vi "Teleop.vi"(10 "Match Info":T1={"Autonomous Elapsed Seconds"=0.0, "TeleOp Elapsed Seconds"=0.0, "Disabled Elapsed Seconds"=0.0, "Visited Autonomous"=FALSE, "Visited TeleOp"=FALSE, "Visited Disabled"=FALSE, "Autonomous Settings"={"Autonomous Style"=enum."Independent", "VI Refnum"=refnum}}, 11 "Call Context":T2) -> ()   [LabVIEW 2012]
doc: "This VI is called for each TeleOp packet received from the DS where the robot is not disabled. It is often used to read from the joysticks and update I/O or to update setpoints for timed control loops. It should complete and return within 20 milliseconds or it may miss DS packets."
uses:
  <vilib>/Rock Robotics/WPI/DriverStation/WPI_DriverStationDerivedRobotMode.ctl
  <vilib>/Rock Robotics/WPI/DriverStation/WPI_DriverStationMatch Info.ctl
  <vilib>/Rock Robotics/WPI/Relay/WPI_RelayValue.ctl
  Robot Global Data.vi
  <vilib>/Rock Robotics/WPI/Joystick/WPI_JoystickGetSetRefNum.vi
panel:
  in  "Ext Const":dbl=0.5
  in  "Dep Const":dbl=1.0
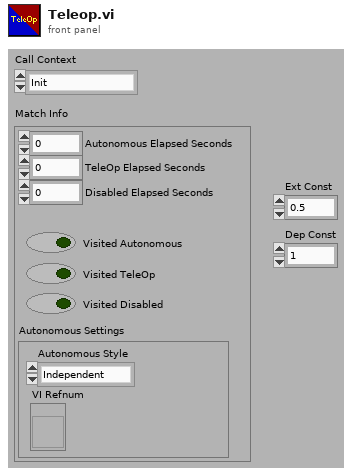
[diagram p1: front panel]
types:
  T1 = typedef "WPI_DriverStationMatch Info.ctl" = cluster{"Autonomous Elapsed Seconds":dbl, "TeleOp Elapsed Seconds":dbl, "Disabled Elapsed Seconds":dbl, "Visited Autonomous":bool, "Visited TeleOp":bool, "Visited Disabled":bool, "Autonomous Settings":cluster{"Autonomous Style":enum16{"Iterative", "Independent"}, "VI Refnum":refnum<vi>}}
  T2 = typedef "WPI_DriverStationDerivedRobotMode.ctl" = enum16{"Init", "Execute", "Stop"}
  T3 = typedef "WPI_RelayValue.ctl" = enum16{"Off", "On", "Forward", "Reverse"}
  T4 = cluster{"Driver Station Digital Input (1-8)[0]":bool, "Driver Station Digital Input (1-8)[1]":bool, "Driver Station Digital Input (1-8)[2]":bool, "Driver Station Digital Input (1-8)[3]":bool, "Driver Station Digital Input (1-8)[4]":bool, "Driver Station Digital Input (1-8)[5]":bool, "Driver Station Digital Input (1-8)[6]":bool, "Driver Station Digital Input (1-8)[7]":bool, "Driver Station Digital Input (1-8)[8]":bool}
  T5 = cluster{"Right Servo High":dbl, "Right Servo Mid":dbl, "Right Servo Low":dbl, "Left Servo High":dbl, "Left Servo Mid":dbl, "Left Servo Low":dbl}
  T6 = typedef "WPI_JoystickDevRef.ctl" = cluster{"Device":T7}
  T7 = typedef "WPI_JoystickDeviceEnum.ctl" = enum16{"USB 1", "USB 2", "USB 3", "USB 4", "Kinect 1", "Kinect 2"}
  T8 = cluster{"axis 1 (x)":dbl, "axis 2 (y)":dbl, "axis 3 (throttle)":dbl, "axis 4":dbl, "axis 5":dbl, "axis 6":dbl}
  T9 = typedef "WPI_RelayDevRef.ctl" = cluster{"DevStatus":errorcluster, "Relay Channel":T10, "Digital Module":T11, "Relay Direction":T12}
  T10 = typedef "FPGA_DIORelayChannel.ctl" = enum8{"Relay 1", "Relay 2", "Relay 3", "Relay 4", "Relay 5", "Relay 6", "Relay 7", "Relay 8", "Invalid"}
  T11 = typedef "FPGA_TypedefDigitalModule.ctl" = enum16{"Digital Module 1", "Digital Module 2"}
  T12 = typedef "WPI_RelayDirection.ctl" = enum16{"Both directions", "Forward only", "Reverse only"}
  T13 = typedef "WPI_ServoDeviceRef.ctl" = cluster{"DeviceStatus":errorcluster, "Digital Module":T11, "PWM Channel":T14, "DeadBand":T15}
  T14 = typedef "FPGA_DIOPWMChannel.ctl" = enum8{"PWM 1", "PWM 2", "PWM 3", "PWM 4", "PWM 5", "PWM 6", "PWM 7", "PWM 8", "PWM 9", "PWM 10", "Invalid"}
  T15 = typedef "WPI_PWMDeadband.ctl" = cluster{"Name":string, "maxPositivePwm":i32, "minPositivePwm":i32, "centerPwm":i32, "maxNegativePwm":i32, "minNegativePwm":i32, "angularRange":u16}
  T16 = typedef "WPI_MotorControlDeviceRef.ctl" = cluster{"DeviceStatus":errorcluster, "Type":enum16{"PWM", "CAN"}, "PWM":cluster{"Digital Module":T11, "PWM Channel":T14, "DeadBand":T15}, "CAN":cluster{"Device Number":u8, "Control Mode":T17, "Semaphore":T18, "Max Vout":dbl}, "Invert":bool, "TransformRef":T19, "InvTransformRef":T19}
  T17 = typedef "WPI_CANJaguar_ControlMode.ctl" = enum8{"Percent VBus", "Current", "Speed", "Position", "Voltage"}
  T18 = typedef "Semaphore RefNum" = refnum<k1>
  T19 = typedef "WPI_PWMTransform_ConPane.ctl" = refnum<vi>
  T20 = typedef "WPI_JoystickButtonState.ctl" = cluster{"Button 1":bool, "Button 2":bool, "Button 3":bool, "Button 4":bool, "Button 5":bool, "Button 6":bool, "Button 7":bool, "Button 8":bool, "Button 9":bool, "Button 10":bool, "Button 11":bool, "Button 12":bool}
  T21 = cluster{"FlipperLeftUp":dbl, "FlipperLeftDown":dbl, "FlipperRightUp":dbl, "FlipperRightDown":dbl, "KickerLeftBack":dbl, "KickerLeftForward":dbl, "KickerRightBack":dbl, "KickerRightForward":dbl}
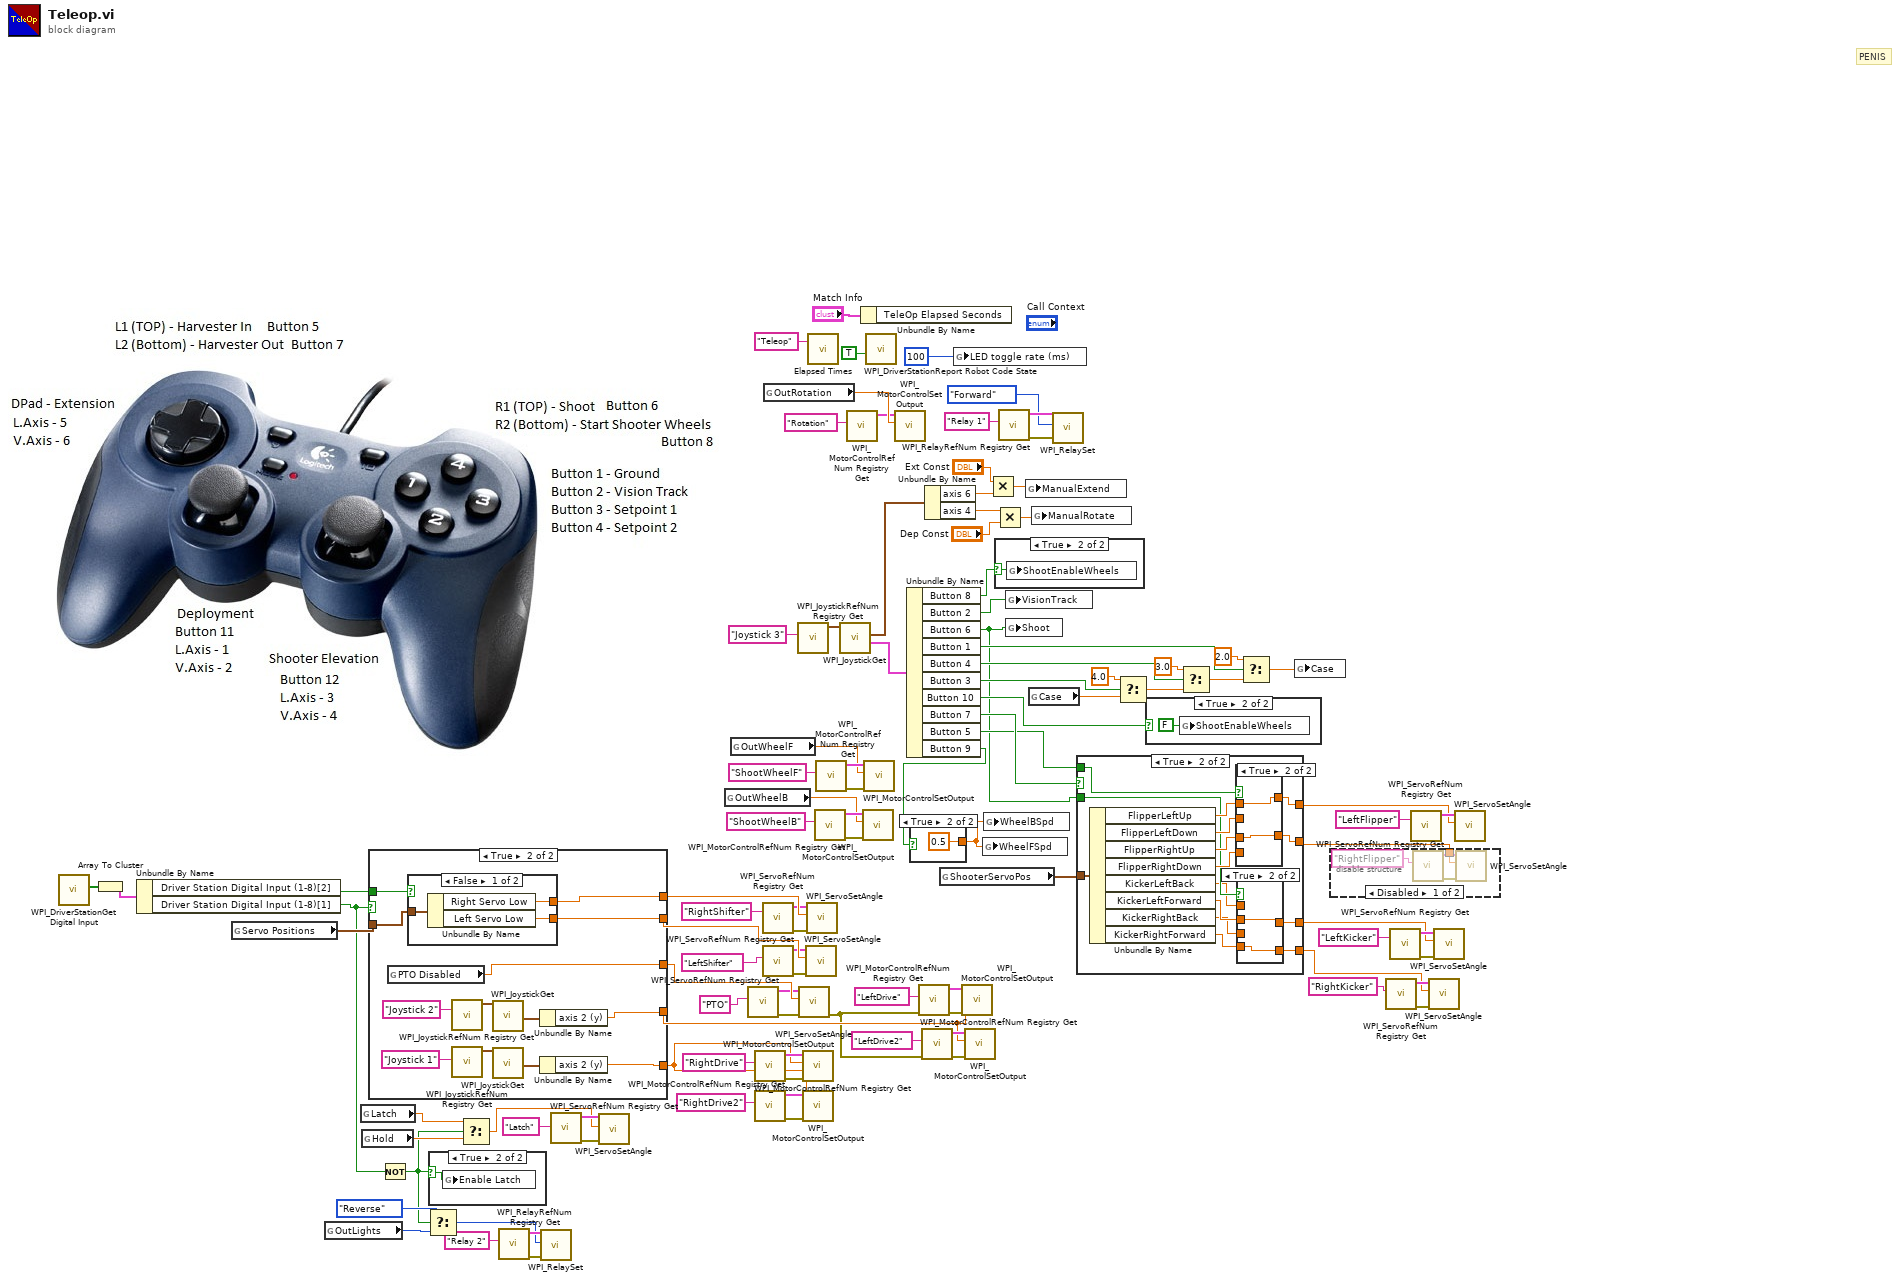
[diagram p0: block diagram]
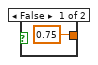
[diagram p2: hidden frame]
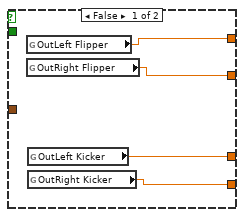
[diagram p4: hidden frame]
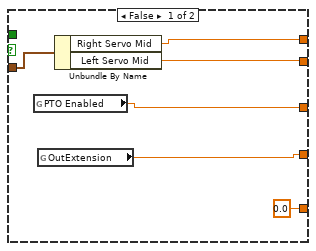
[diagram p8: hidden frame]
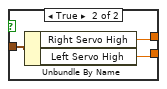
[diagram p9: hidden frame]
diagram:
  # "PENIS"
  n1 = call <vilib>:"WPI_DriverStationGet Digital Input.vi"() -> ("Driver Station Digital Input (1-8)"=w73:bool[])  [unwired: 11 in]
  n2 = Array To Cluster(array=w73) -> (cluster=w72:T4)
  n3 = Unbundle By Name(w72) -> ("Driver Station Digital Input (1-8)[2]"=w71:bool, "Driver Station Digital Input (1-8)[1]"=w32:bool)
  n4 = global read "Robot Global Data.vi" "Servo Positions"() -> (w70:T5)
  n5 = global read "Robot Global Data.vi" "OutLights"() -> (w38:T3)
  n6 = global read "Robot Global Data.vi" "Latch"() -> (w5:dbl)
  n7 = global read "Robot Global Data.vi" "Hold"() -> (w4:dbl)
  n8 = case shown="True" w32 {
    tunnel: w71 -> [_ w124]
    tunnel: w70 -> [w111 w123]
    tunnel: [w110 w122] -> w69
    tunnel: [w109 w121] -> w68
    tunnel: [w108 w120] -> w61
    tunnel: [w106 w113] -> w60
    tunnel: [0.0 w112] -> w59
    frame False {
      n9 = global read "Robot Global Data.vi" "PTO Enabled"() -> (w108:dbl)
      n10 = global read "Robot Global Data.vi" "OutExtension"() -> (w106:dbl)
      n11 = Unbundle By Name(w111) -> ("Right Servo Mid"=w110:dbl, "Left Servo Mid"=w109:dbl)
    }
    frame True {
      n12 = global read "Robot Global Data.vi" "PTO Disabled"() -> (w120:dbl)
      n13 = case shown="False" w124 {
        tunnel: w123 -> [w127 w130]
        tunnel: [w126 w129] -> w122
        tunnel: [w125 w128] -> w121
        frame False {
          n14 = Unbundle By Name(w127) -> ("Right Servo Low"=w126:dbl, "Left Servo Low"=w125:dbl)
        }
        frame True {
          n15 = Unbundle By Name(w130) -> ("Right Servo High"=w129:dbl, "Left Servo High"=w128:dbl)
        }
      }
      n16 = call <vilib>:"WPI_JoystickRefNum Registry Get.vi"("refnum name"="Joystick 2") -> ("JoystickDevRef"=w114:T6)  [unwired: 1 in, 9 out]
      n17 = call <vilib>:"WPI_JoystickRefNum Registry Get.vi"("refnum name"="Joystick 1") -> ("JoystickDevRef"=w118:T6)  [unwired: 1 in, 9 out]
      n18 = call <vilib>:"WPI_JoystickGet.vi"("JoystickDevRef"=w114) -> ("Axes"=w116:T8)  [unwired: 1 in, 5 out]
      n19 = call <vilib>:"WPI_JoystickGet.vi"("JoystickDevRef"=w118) -> ("Axes"=w119:T8)  [unwired: 1 in, 5 out]
      n20 = Unbundle By Name(w116) -> ("axis 2 (y)"=w113:dbl)
      n21 = Unbundle By Name(w119) -> ("axis 2 (y)"=w112:dbl)
    }
  }
  n22 = Not(x=w32) -> (.not. x?=w3:bool)
  n23 = Select(t=WPI_RelayValue."Reverse" ("RelayValue"), s=w3, f=w38) -> (s? t:f=w36:T3)
  n24 = case shown="True" w3 {
    selector: w3 -> [_ w131]
    frame False {
    }
    frame True {
      n25 = global write "Robot Global Data.vi" "Enable Latch"(w131) -> ()
    }
  }
  n26 = Select(t=w5, s=w3, f=w4) -> (s? t:f=w31:dbl)
  n27 = call <vilib>:"WPI_RelayRefNum Registry Get.vi"("refnum name"="Relay 2") -> ("error out"=w44:errorcluster, "RelayDevRef"=w42:T9)  [unwired: 9 in]
  n28 = call <vilib>:"WPI_RelaySet.vi"("error in (no error)"=w44, "RelayValue"=w36, "RelayDevRef"=w42) -> ()  [unwired: 7 in, 2 out]
  n29 = call <vilib>:"WPI_ServoRefNum Registry Get.vi"("refnum name"="Latch") -> ("error out"=w35:errorcluster, "ServoDeviceRef"=w33:T13)  [unwired: 9 in]
  n30 = call <vilib>:"WPI_ServoSetAngle.vi"("error in (no error)"=w35, "Angle"=w31, "ServoDeviceRef"=w33) -> ()  [unwired: 7 in, 2 out]
  n31 = global read "Robot Global Data.vi" "OutWheelB"() -> (w23:dbl)
  n32 = global read "Robot Global Data.vi" "OutWheelF"() -> (w24:dbl)
  n33 = call <vilib>:"WPI_ServoRefNum Registry Get.vi"("refnum name"="PTO") -> ("error out"=w54:errorcluster, "ServoDeviceRef"=w55:T13)  [unwired: 9 in]
  n34 = call <vilib>:"WPI_MotorControlRefNum Registry Get.vi"("refnum name"="RightDrive") -> ("error out"=w83:errorcluster, "MotorControlDevRef"=w85:T16)  [unwired: 9 in]
  n35 = call <vilib>:"WPI_MotorControlRefNum Registry Get.vi"("refnum name"="RightDrive2") -> ("error out"=w76:errorcluster, "MotorControlDevRef"=w74:T16)  [unwired: 9 in]
  n36 = call <vilib>:"WPI_ServoRefNum Registry Get.vi"("refnum name"="RightShifter") -> ("error out"=w64:errorcluster, "ServoDeviceRef"=w65:T13)  [unwired: 9 in]
  n37 = call <vilib>:"WPI_ServoRefNum Registry Get.vi"("refnum name"="LeftShifter") -> ("error out"=w66:errorcluster, "ServoDeviceRef"=w67:T13)  [unwired: 9 in]
  n38 = global read "Robot Global Data.vi" "OutRotation"() -> (w58:dbl)
  n39 = call <vilib>:"WPI_JoystickRefNum Registry Get.vi"("refnum name"="Joystick 3") -> ("JoystickDevRef"=w102:T6)  [unwired: 9 in, 1 out]
  n40 = call <vilib>:"WPI_ServoSetAngle.vi"("error in (no error)"=w54, "Angle"=w61, "ServoDeviceRef"=w55) -> ("error out"=w50:errorcluster)  [unwired: 7 in, 1 out]
  n41 = call <vilib>:"WPI_MotorControlSetOutput.vi"("error in (no error)"=w83, "Output"=w59, "MotorControlDevRef"=w85) -> ()  [unwired: 6 in, 3 out]
  n42 = call <vilib>:"WPI_MotorControlSetOutput.vi"("error in (no error)"=w76, "Output"=w59, "MotorControlDevRef"=w74) -> ()  [unwired: 6 in, 3 out]
  n43 = call <vilib>:"WPI_ServoSetAngle.vi"("error in (no error)"=w66, "Angle"=w68, "ServoDeviceRef"=w67) -> ()  [unwired: 7 in, 2 out]
  n44 = call <vilib>:"WPI_ServoSetAngle.vi"("error in (no error)"=w64, "Angle"=w69, "ServoDeviceRef"=w65) -> ()  [unwired: 7 in, 2 out]
  n45 = call "Elapsed Times.vi"("Call Name"="Teleop") -> ()  [unwired: 2 in, 1 out]
  n46 = call <vilib>:"WPI_MotorControlRefNum Registry Get.vi"("refnum name"="ShootWheelB") -> ("error out"=w26:errorcluster, "MotorControlDevRef"=w27:T16)  [unwired: 9 in]
  n47 = call <vilib>:"WPI_MotorControlRefNum Registry Get.vi"("refnum name"="ShootWheelF") -> ("error out"=w28:errorcluster, "MotorControlDevRef"=w25:T16)  [unwired: 9 in]
  n48 = call <vilib>:"WPI_JoystickGet.vi"("JoystickDevRef"=w102) -> ("Buttons"=w100:T20, "Axes"=w99:T8)  [unwired: 4 in, 1 out]
  n49 = call <vilib>:"WPI_MotorControlRefNum Registry Get.vi"("refnum name"="Rotation") -> ("MotorControlDevRef"=w56:T16)  [unwired: 9 in, 1 out]
  n50 = Unbundle By Name("Match Info") -> ()  [unwired: 1 out]
  n51 = call <vilib>:"WPI_MotorControlSetOutput.vi"("error in (no error)"=w26, "Output"=w23, "MotorControlDevRef"=w27) -> ()  [unwired: 6 in, 3 out]
  n52 = call <vilib>:"WPI_MotorControlSetOutput.vi"("error in (no error)"=w28, "Output"=w24, "MotorControlDevRef"=w25) -> ()  [unwired: 6 in, 3 out]
  n53 = call <vilib>:"WPI_DriverStationReport Robot Code State.vi"("TeleOp"=TRUE ("Autonomous")) -> ()  [unwired: 10 in, 1 out]
  n54 = call <vilib>:"WPI_MotorControlSetOutput.vi"("Output"=w58, "MotorControlDevRef"=w56) -> ()  [unwired: 7 in, 3 out]
  n55 = Unbundle By Name(w100) -> ("Button 8"=w87:bool, "Button 2"=w98:bool, "Button 6"=w7:bool, "Button 1"=w97:bool, "Button 4"=w95:bool, "Button 3"=w94:bool, "Button 10"=w22:bool, "Button 7"=w21:bool, "Button 5"=w20:bool, "Button 9"=w1:bool)
  n56 = case shown="True" w1 {
    tunnel: [0.75 0.5] -> w2
    frame False {
    }
    frame True {
    }
  }
  n57 = call <vilib>:"WPI_MotorControlRefNum Registry Get.vi"("error in (no error)"=w50, "refnum name"="LeftDrive") -> ("error out"=w78:errorcluster, "MotorControlDevRef"=w81:T16)  [unwired: 8 in]
  n58 = call <vilib>:"WPI_MotorControlRefNum Registry Get.vi"("error in (no error)"=w50, "refnum name"="LeftDrive2") -> ("error out"=w77:errorcluster, "MotorControlDevRef"=w79:T16)  [unwired: 8 in]
  n59 = Unbundle By Name(w99) -> ("axis 6"=w41:dbl, "axis 4"=w51:dbl)
  n60 = global read "Robot Global Data.vi" "ShooterServoPos"() -> (w8:T21)
  n61 = global write "Robot Global Data.vi" "LED toggle rate (ms)"(u32 100 ("LED ms toggle rate")) -> ()
  n62 = call <vilib>:"WPI_MotorControlSetOutput.vi"("error in (no error)"=w78, "Output"=w60, "MotorControlDevRef"=w81) -> ()  [unwired: 6 in, 3 out]
  n63 = call <vilib>:"WPI_MotorControlSetOutput.vi"("error in (no error)"=w77, "Output"=w60, "MotorControlDevRef"=w79) -> ()  [unwired: 6 in, 3 out]
  n64 = global write "Robot Global Data.vi" "WheelFSpd"(w2) -> ()
  n65 = global write "Robot Global Data.vi" "WheelBSpd"(w2) -> ()
  n66 = Multiply(x="Ext Const", y=w41) -> (x*y=w39:dbl)
  n67 = Multiply(x=w51, y="Dep Const") -> (x*y=w49:dbl)
  n68 = case shown="True" w87 {
    selector: w87 -> [_ w134]
    frame False {
    }
    frame True {
      n69 = global write "Robot Global Data.vi" "ShootEnableWheels"(w134) -> ()
    }
  }
  n70 = call <vilib>:"WPI_RelayRefNum Registry Get.vi"("refnum name"="Relay 1") -> ("error out"=w46:errorcluster, "RelayDevRef"=w48:T9)  [unwired: 9 in]
  n71 = global write "Robot Global Data.vi" "VisionTrack"(w98) -> ()
  n72 = global write "Robot Global Data.vi" "Shoot"(w7) -> ()
  n73 = global write "Robot Global Data.vi" "ManualExtend"(w39) -> ()
  n74 = global read "Robot Global Data.vi" "Case"() -> (w89:dbl)
  n75 = global write "Robot Global Data.vi" "ManualRotate"(w49) -> ()
  n76 = call <vilib>:"WPI_RelaySet.vi"("error in (no error)"=w46, "RelayValue"=WPI_RelayValue."Forward", "RelayDevRef"=w48) -> ()  [unwired: 7 in, 2 out]
  n77 = case shown="True" w21 {
    tunnel: w20 -> [_ w139]
    tunnel: [w138 w152] -> w11
    tunnel: [w137 w150] -> w10
    tunnel: [w136 w141] -> w9
    tunnel: [w135 w140] -> w6
    tunnel: w8 -> [_ w153]
    tunnel: w7 -> [_ w146]
    frame False {
      n78 = global read "Robot Global Data.vi" "OutLeft Flipper"() -> (w138:dbl)
      n79 = global read "Robot Global Data.vi" "OutRight Flipper"() -> (w137:dbl)
      n80 = global read "Robot Global Data.vi" "OutLeft Kicker"() -> (w136:dbl)
      n81 = global read "Robot Global Data.vi" "OutRight Kicker"() -> (w135:dbl)
    }
    frame True {
      n82 = Unbundle By Name(w153) -> ("FlipperLeftUp"=w151:dbl, "FlipperLeftDown"=w148:dbl, "FlipperRightUp"=w149:dbl, "FlipperRightDown"=w147:dbl, "KickerLeftBack"=w145:dbl, "KickerLeftForward"=w144:dbl, "KickerRightBack"=w143:dbl, "KickerRightForward"=w142:dbl)
      n83 = case shown="True" w139 {
        tunnel: [w159 w161] -> w152
        tunnel: w151 -> [_ w161]
        tunnel: [w158 w160] -> w150
        tunnel: w149 -> [_ w160]
        tunnel: w148 -> [w159 _]
        tunnel: w147 -> [w158 _]
        frame False {
        }
        frame True {
        }
      }
      n84 = case shown="True" w146 {
        tunnel: w145 -> [w155 _]
        tunnel: w144 -> [_ w156]
        tunnel: w143 -> [w154 _]
        tunnel: w142 -> [_ w157]
        tunnel: [w155 w156] -> w141
        tunnel: [w154 w157] -> w140
        frame False {
        }
        frame True {
        }
      }
    }
  }
  n85 = Select(t=4.0, s=w94, f=w89) -> (s? t:f=w93:dbl)
  n86 = case shown="True" w22 {
    frame False {
    }
    frame True {
      n87 = global write "Robot Global Data.vi" "ShootEnableWheels"(FALSE ("ShootStartWheels")) -> ()
    }
  }
  n88 = Select(t=3.0, s=w95, f=w93) -> (s? t:f=w91:dbl)
  n89 = Select(t=2.0, s=w97, f=w91) -> (s? t:f=w88:dbl)
  n90 = global write "Robot Global Data.vi" "Case"(w88) -> ()
  n91 = disable-structure shown="Disabled" {
    disable-tunnel: w10 -> [w163 _]
    frame Disabled {
      n92 = call <vilib>:"WPI_ServoRefNum Registry Get.vi"("refnum name"="RightFlipper") -> ("error out"=w166:errorcluster, "ServoDeviceRef"=w164:T13)  [unwired: 9 in]
      n93 = call <vilib>:"WPI_ServoSetAngle.vi"("error in (no error)"=w166, "Angle"=w163, "ServoDeviceRef"=w164) -> ()  [unwired: 7 in, 2 out]
    }
    frame Enabled {
    }
  }
  n94 = call <vilib>:"WPI_ServoRefNum Registry Get.vi"("refnum name"="RightKicker") -> ("error out"=w18:errorcluster, "ServoDeviceRef"=w16:T13)  [unwired: 9 in]
  n95 = call <vilib>:"WPI_ServoRefNum Registry Get.vi"("refnum name"="LeftKicker") -> ("error out"=w12:errorcluster, "ServoDeviceRef"=w13:T13)  [unwired: 9 in]
  n96 = call <vilib>:"WPI_ServoRefNum Registry Get.vi"("refnum name"="LeftFlipper") -> ("ServoDeviceRef"=w14:T13)  [unwired: 9 in, 1 out]
  n97 = call <vilib>:"WPI_ServoSetAngle.vi"("error in (no error)"=w18, "Angle"=w6, "ServoDeviceRef"=w16) -> ()  [unwired: 7 in, 2 out]
  n98 = call <vilib>:"WPI_ServoSetAngle.vi"("error in (no error)"=w12, "Angle"=w9, "ServoDeviceRef"=w13) -> ()  [unwired: 7 in, 2 out]
  n99 = call <vilib>:"WPI_ServoSetAngle.vi"("Angle"=w11, "ServoDeviceRef"=w14) -> ()  [unwired: 8 in, 2 out]
